vi "Tone Glide Method Comparison.vi"() -> ()   [LabVIEW 2015]
uses:
  Waveform VIs/Tone VIs/Tone Params.ctl
panel:
  out "Waveform Graph":dbl[][](graph)
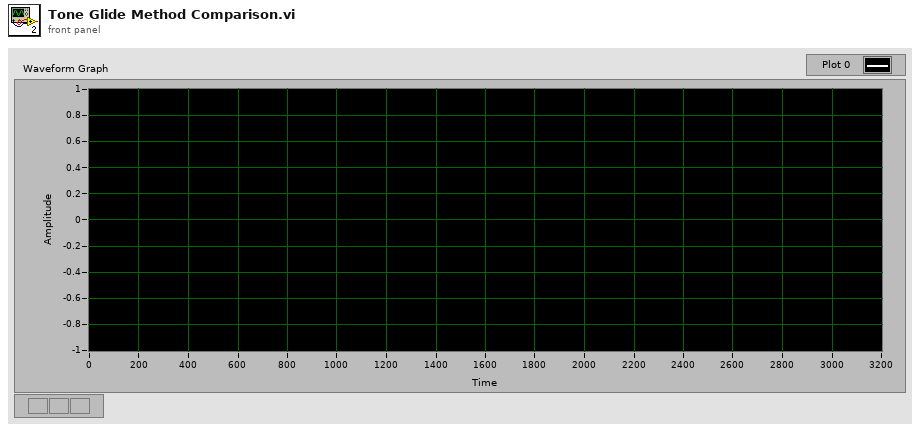
[diagram p1: front panel]
types:
  T1 = typedef "Tone Params.ctl" = cluster{"Frequency (kHz)":dbl, "Last Freq":dbl, "Last Phase":dbl}
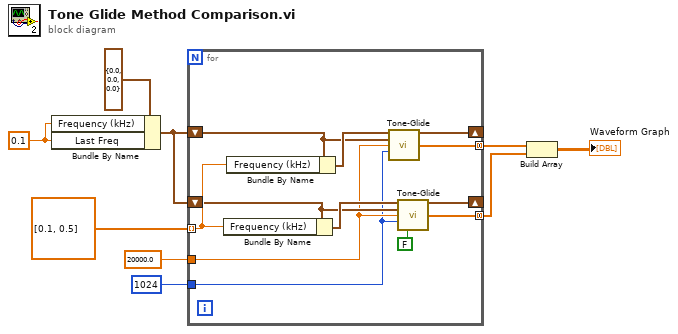
[diagram p0: block diagram]
diagram:
  w8 = 0.1
  n1 = Bundle By Name(cluster=T1 {"Frequency (kHz)"=0.0, "Last Freq"=0.0, "Last Phase"=0.0} ("New"), "Frequency (kHz)"=w8, "Last Freq"=w8) -> (w4:T1)
  n2 = for {
    shift-right: [w21] -> _
    shift-left: w4 -> [w19]
    tunnel: dbl[] [0.1, 0.5] -> [w16] mode=indexing
    tunnel: 20000.0 -> [w13]
    tunnel: 1024 -> [w12]
    tunnel: [w18] -> w1 mode=concatenating
    shift-right: [w17] -> _
    shift-left: w4 -> [w14]
    tunnel: [w10] -> w3 mode=concatenating
    n3 = Bundle By Name(cluster=w14, "Frequency (kHz)"=w16) -> (w15:T1)
    n4 = Bundle By Name(cluster=w19, "Frequency (kHz)"=w16) -> (w20:T1)
    n5 = call "Tone-Glide.vi"("New"=w20, "Old"=w19, "Fs (Hz)"=w13, "Npts"=w12) -> ("Params out"=w21:T1, "Y"=w18:dbl[])  [unwired: 10 in]
    n6 = call "Tone-Glide.vi"("New"=w15, "Old"=w14, "Fs (Hz)"=w13, "Npts"=w12, "Original method?"=FALSE) -> ("Params out"=w17:T1, "Y"=w10:dbl[])  [unwired: 9 in]
  }
  n7 = Build Array(w1, w3) -> (→"Waveform Graph":dbl[][])
